vi "查询clonm对应的所有内容.vi"(7 "条件":enum16{"DISTINCT", "MIN", "MAX"}(ring), 8 "error in (no error)":errorcluster caption="错误输入（无错误）", 9 "组合框":string(combo), 10 "database":string="database1.mdb", 11 "table":string(combo)="CODMn") -> (0 "error out":errorcluster caption="错误输出", 3 "输出数组":string[](array[string]))   [LabVIEW 2016]
uses:
  <vilib>/Utility/sysdir.llb/System Directory Type.ctl
  <vilib>/addons/database/Connection.llb/DB Tools Open Connec (String).vi
  <vilib>/addons/database/Connection.llb/Conn Execute.vi
  <vilib>/addons/database/Recordset.llb/Rec Fetch Recordset Data (R).vi
  <vilib>/addons/database/Recordset.llb/Rec Destroy - Connection.vi
  <vilib>/addons/database/_DB Variant To Data/Database Variant To Data.xnode
  <vilib>/addons/database/NI_Database_API.lvlib
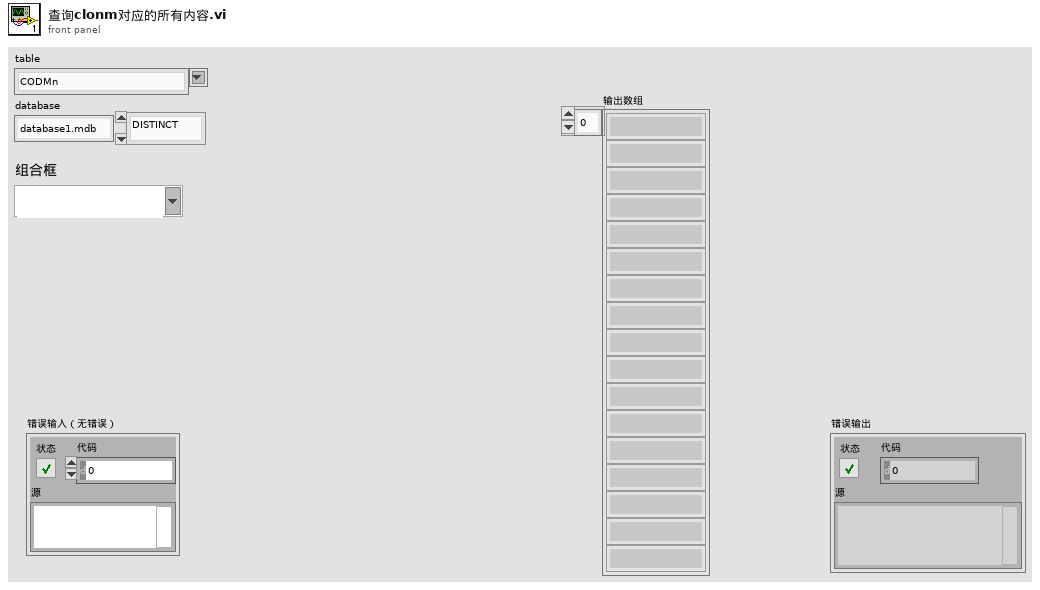
[diagram p1: front panel]
types:
  T1 = typedef "System Directory Type.ctl" = i32
  T2 = typedef "NI_Database_API.lvlib/Conn ObjectReference.ctl" = refnum<k1>
  T3 = typedef "NI_Database_API.lvlib/Rec ObjectReference.ctl" = refnum<k1>
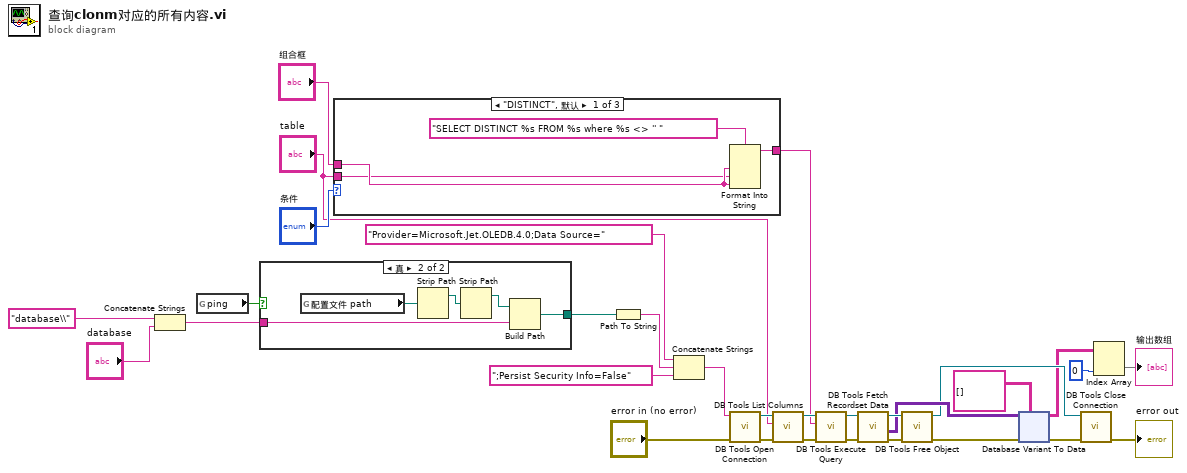
[diagram p0: block diagram]
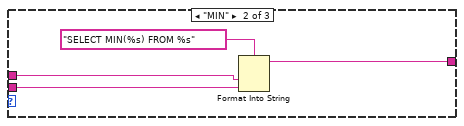
[diagram p2: hidden frame]
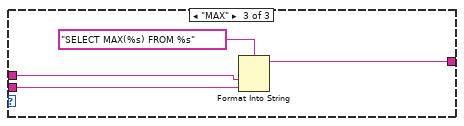
[diagram p3: hidden frame]
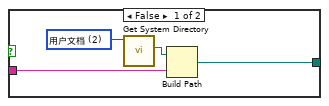
[diagram p4: hidden frame]
diagram:
  n1 = Concatenate Strings("database\\" ("名称或相对路径"), "database") -> (w23:string)
  n2 = global read "ping全局.vi" "ping"() -> (w24:bool)
  n3 = case shown="真" w24 {
    tunnel: w23 -> [w33 w39]
    tunnel: [w32 w37] -> w22
    frame False {
      w34 = T1 2 items=["用户目录"=0, "用户桌面"=1, "用户文档"=2, "用户应用程序数据"=3, "用户设置"=4, "用户临时目录"=5, "公共文档"=6, "公共应用程序数据"=7, "公共设置"=8, "公共缓存"=13, "系统核心库"=9, "系统安装库"=10, "应用程序文件"=11, "启动盘根目录"=12] ("system directory type")
      n4 = call <vilib>:"Get System Directory.vi"("system directory type"=w34) -> ("system directory"=w35:path)  [unwired: 10 in]
      n5 = Build Path(base path=w35, name or relative path=w33) -> (appended path=w32:path)
    }
    frame True {
      n6 = global read "ping全局.vi" "配置文件 path"() -> (w36:path)
      n7 = Strip Path(path=w36) -> (stripped path=w40:path)  [unwired: 1 out]
      n8 = Strip Path(path=w40) -> (stripped path=w38:path)  [unwired: 1 out]
      n9 = Build Path(base path=w38, name or relative path=w39) -> (appended path=w37:path)
    }
  }
  n10 = case shown="\"DISTINCT\", 默认" "条件" {
    tunnel: [w44 w45 w49] -> w2
    tunnel: "组合框" -> [w42 w46 w51]
    tunnel: "table" -> [w41 w47 w50]
    frame "DISTINCT", Default {
      n11 = Format Into String(format string="SELECT DISTINCT %s FROM %s where %s <> '' ", w42, w41, w42) -> (resulting string=w44:string)  [unwired: 2 in, 1 out]
    }
    frame "MIN" {
      n12 = Format Into String(format string="SELECT MIN(%s) FROM %s", w46, w47) -> (resulting string=w45:string)  [unwired: 2 in, 1 out]
    }
    frame "MAX" {
      n13 = Format Into String(format string="SELECT MAX(%s) FROM %s", w51, w50) -> (resulting string=w49:string)  [unwired: 2 in, 1 out]
    }
  }
  n14 = Path To String(path=w22) -> (string=w27:string)
  n15 = Concatenate Strings("Provider=Microsoft.Jet.OLEDB.4.0;Data Source=", w27, ";Persist Security Info=False") -> (w20:string)
  n16 = call-poly <vilib>:"DB Tools Open Connection.vi"("error in (no error)"="error in (no error)", "connection information"=w20) -> ("error out"=w30:errorcluster, "connection reference"=w31:T2)  [unwired: 6 in]
  n17 = call <vilib>:"DB Tools List Columns.vi"("error in (no error)"=w30, "table"="table", "connection reference"=w31) -> ("error out"=w8:errorcluster, "connection reference out"=w9:T2)  [unwired: 1 in, 2 out]
  n18 = call-poly <vilib>:"DB Tools Execute Query.vi"("error in (no error)"=w8, "SQL query"=w2, "connection reference"=w9) -> ("error out"=w18:errorcluster, "recordset reference"=w19:T3)  [unwired: 5 in]
  n19 = call-poly <vilib>:"DB Tools Fetch Recordset Data.vi"("error in (no error)"=w18, "recordset reference"=w19) -> ("error out"=w17:errorcluster, "recordset data"=w13:variant[][], "recordset reference out"=w16:T3)  [unwired: 3 in]
  n20 = call-poly <vilib>:"DB Tools Free Object.vi"("error in (no error)"=w17, "recordset reference"=w16) -> ("error out"=w12:errorcluster, "connection reference"=w11:T2)  [unwired: 8 in]
  n21 = xnode "Database Variant To Data"("database variant"=w13, "error in (no error)"=w12, "type"=string[][] []) -> ("data"=w7:string[][], "error out"=w14:errorcluster)
  n22 = call <vilib>:"DB Tools Close Connection.vi"("error in (no error)"=w14, "connection reference"=w11) -> ("error out"=→"error out":errorcluster)  [unwired: 5 in]
  n23 = Index Array(array=w7, index (col)=0 ("禁用的索引 (列)")) -> (element=→"输出数组":string[])  [unwired: 1 in]
